vi "Read Target Project Path.vi"(8 "error in (no error)":errorcluster, 11 "RIO Target Configuration in":refnum<class "RIO Target Configuration.lvclass">) -> (0 "error out":errorcluster, 2 "Target Project Path":path, 3 "RIO Target Configuration out":refnum<class "RIO Target Configuration.lvclass">)   [LabVIEW 2014, in "RIO Target Configuration.lvclass"]
uses:
  RIO Target Configuration.lvclass
  RIO Target Configuration.lvclass/RIO Target Configuration.ctl
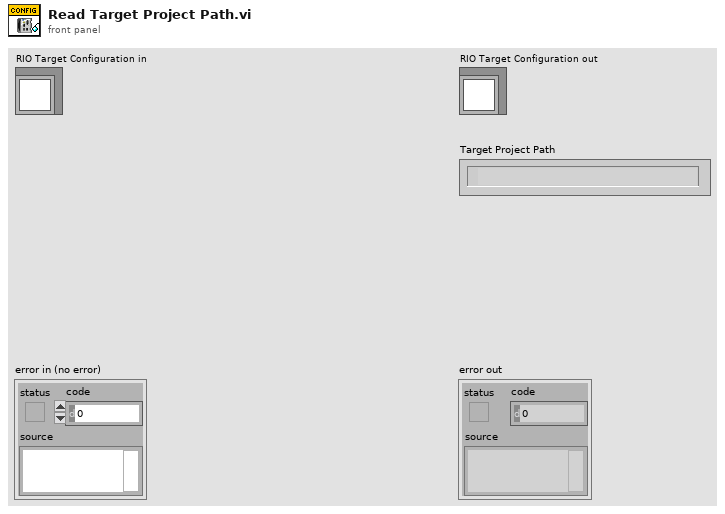
[diagram p1: front panel]
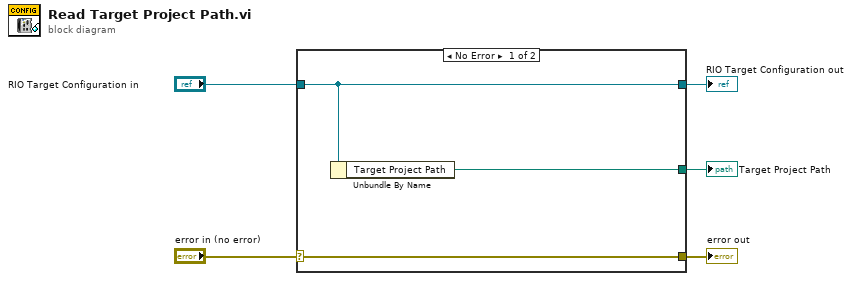
[diagram p0: block diagram]
diagram:
  n1 = case shown="No Error" "error in (no error)" {
    selector: "error in (no error)" -> [w8 w9]
    tunnel: [w8 w9] -> w4
    tunnel: [w7 w10] -> w2
    tunnel: "RIO Target Configuration in" -> [w7 w10]
    tunnel: [w6 _] -> w1
    frame No Error {
      n2 = Unbundle By Name(w7) -> ("Target Project Path"=w6:path)
    }
    frame Error {
    }
  }
  "error out" <- w4
  "RIO Target Configuration out" <- w2
  "Target Project Path" <- w1
